vi "Update Gain.vi"(8 "error in (no error)":errorcluster caption="entrée d'erreur (pas d'erreur)", 9 "Gain":dbl, 10 "IMAQdx Session in":T1, 11 "Acq Cam Basler en entrée":refnum<class "Acq Cam Basler.lvclass">) -> (0 "error out":errorcluster caption="sortie d'erreur", 2 "IMAQdx Session out":T1, 3 "Acq Cam Basler en sortie":refnum<class "Acq Cam Basler.lvclass">)   [LabVIEW 2023, in "Acq Cam Basler.lvclass"]
uses:
  Acq Cam Basler.lvclass
  <vilib>/userDefined/High Color/IMAQdx.ctl
  Acq Cam Basler.lvclass/Acq Cam Basler.ctl
  <vilib>/Utility/error.llb/Error Cluster From Error Code.vi
  <vilib>/ErrorRing/Error Ring.xnode
  <resource>/objmgr/imaqdx.rc
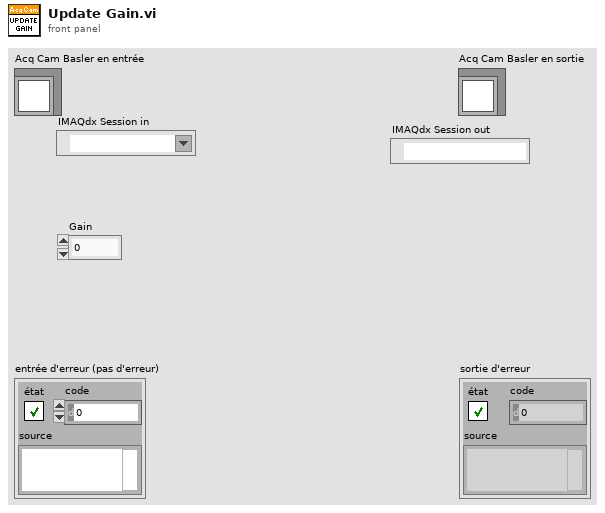
[diagram p1: front panel]
types:
  T1 = typedef "IMAQdx.ctl" = refnum<k21>
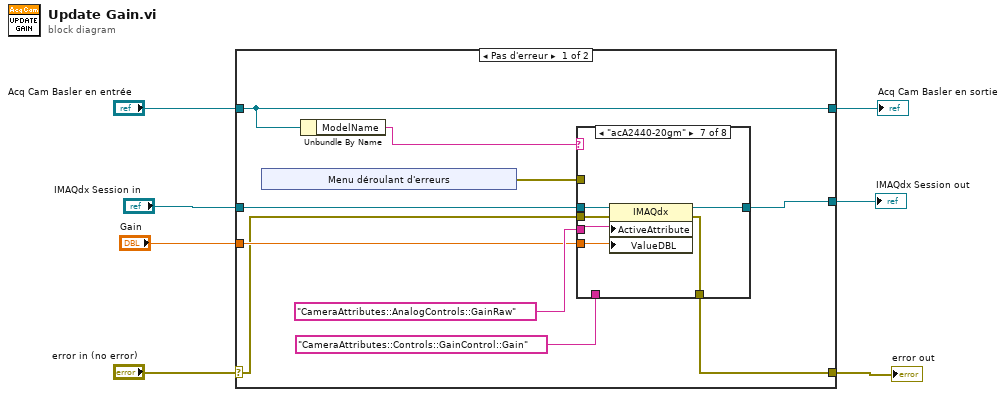
[diagram p0: block diagram]
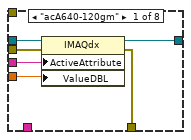
[diagram p2: hidden frame]
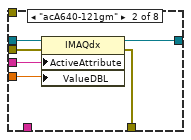
[diagram p3: hidden frame]
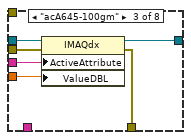
[diagram p4: hidden frame]
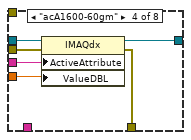
[diagram p5: hidden frame]
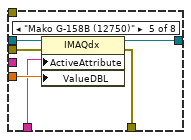
[diagram p6: hidden frame]
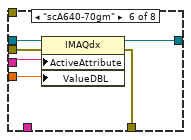
[diagram p7: hidden frame]
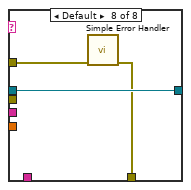
[diagram p8: hidden frame]
diagram:
  n1 = case shown="Pas d'erreur" "error in (no error)" {
    selector: "error in (no error)" -> [w15 w70]
    tunnel: [w14 w70] -> w6
    tunnel: [w11 w69] -> w4
    tunnel: "Acq Cam Basler en entrée" -> [w11 w69]
    tunnel: "Gain" -> [w16 _]
    tunnel: [w13 w68] -> w2
    tunnel: "IMAQdx Session in" -> [w12 w68]
    frame No Error {
      n2 = xnode "Menu déroulant d'erreurs"() -> ("sortie d'erreur"=w9:errorcluster)
      n3 = Unbundle By Name(w11) -> ("ModelName"=w10:string)
      n4 = case shown="\"acA2440-20gm\"" w10 {
        tunnel: "CameraAttributes::AnalogControls::GainRaw" ("ActiveAttribute") -> [w28 w34 w40 w46 _ w53 w59 _]
        tunnel: w16 -> [w27 w33 w39 w45 w52 w58 w64 _]
        tunnel: w15 -> [w26 w32 w38 w44 w51 w57 w63 _]
        tunnel: [w25 w31 w37 w43 w50 w56 w62 w65] -> w14
        tunnel: [w24 w30 w36 w42 w49 w55 w61 w67] -> w13
        tunnel: w12 -> [w23 w29 w35 w41 w48 w54 w60 w67]
        tunnel: w9 -> [_ _ _ _ _ _ _ w66]
        tunnel: "CameraAttributes::Controls::GainControl::Gain" -> [_ _ _ _ w47 _ _ _]
        frame "acA640-120gm" {
          n5 = property class="IMAQdx"(reference=w23, error in=w26, "ActiveAttribute"=w28, "ValueDBL"=w27) -> (reference out=w24:T1, error out=w25:errorcluster)
        }
        frame "acA640-121gm" {
          n6 = property class="IMAQdx"(reference=w29, error in=w32, "ActiveAttribute"=w34, "ValueDBL"=w33) -> (reference out=w30:T1, error out=w31:errorcluster)
        }
        frame "acA645-100gm" {
          n7 = property class="IMAQdx"(reference=w35, error in=w38, "ActiveAttribute"=w40, "ValueDBL"=w39) -> (reference out=w36:T1, error out=w37:errorcluster)
        }
        frame "acA1600-60gm" {
          n8 = property class="IMAQdx"(reference=w41, error in=w44, "ActiveAttribute"=w46, "ValueDBL"=w45) -> (reference out=w42:T1, error out=w43:errorcluster)
        }
        frame "Mako G-158B (12750)" {
          n9 = property class="IMAQdx"(reference=w48, error in=w51, "ActiveAttribute"=w47, "ValueDBL"=w52) -> (reference out=w49:T1, error out=w50:errorcluster)
        }
        frame "scA640-70gm" {
          n10 = property class="IMAQdx"(reference=w54, error in=w57, "ActiveAttribute"=w53, "ValueDBL"=w58) -> (reference out=w55:T1, error out=w56:errorcluster)
        }
        frame "acA2440-20gm" {
          n11 = property class="IMAQdx"(reference=w60, error in=w63, "ActiveAttribute"=w59, "ValueDBL"=w64) -> (reference out=w61:T1, error out=w62:errorcluster)
        }
        frame Default {
          n12 = call <vilib>:"Simple Error Handler.vi"("error in (no error)"=w66) -> ("error out"=w65:errorcluster)  [unwired: 4 in, 4 out]
        }
      }
    }
    frame Error {
    }
  }
  "error out" <- w6
  "Acq Cam Basler en sortie" <- w4
  "IMAQdx Session out" <- w2
